vi "Convert Library and Other Files.vi"(8 "error in":errorcluster, 9 "main module path":path, 10 "project:open":refnum<vi>, 11 "dependency list[]":path[](array[path])) -> (0 "error out":errorcluster, 2 "outside vis":string[](array[string]), 3 "destination directory":path)   [LabVIEW 2021, in "Converter.lvlib"]
uses:
  Converter.lvlib
  TypeDefs/Library Data.ctl
  Converter Reusables/Converter Reusables.lvlib
  Path Functions/Path Functions.lvlib
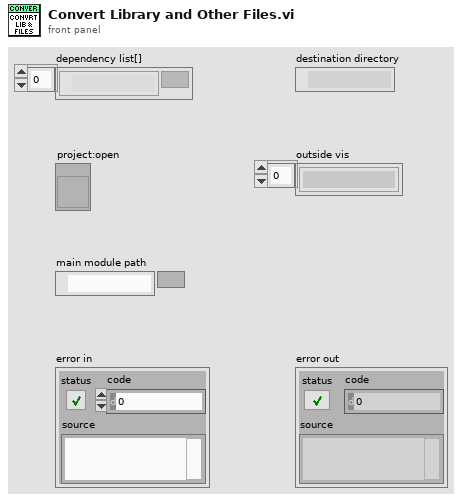
[diagram p1: front panel]
types:
  T1 = typedef "Converter.lvlib/Library Data.ctl" = cluster{"lib path":path, "lib name":string}
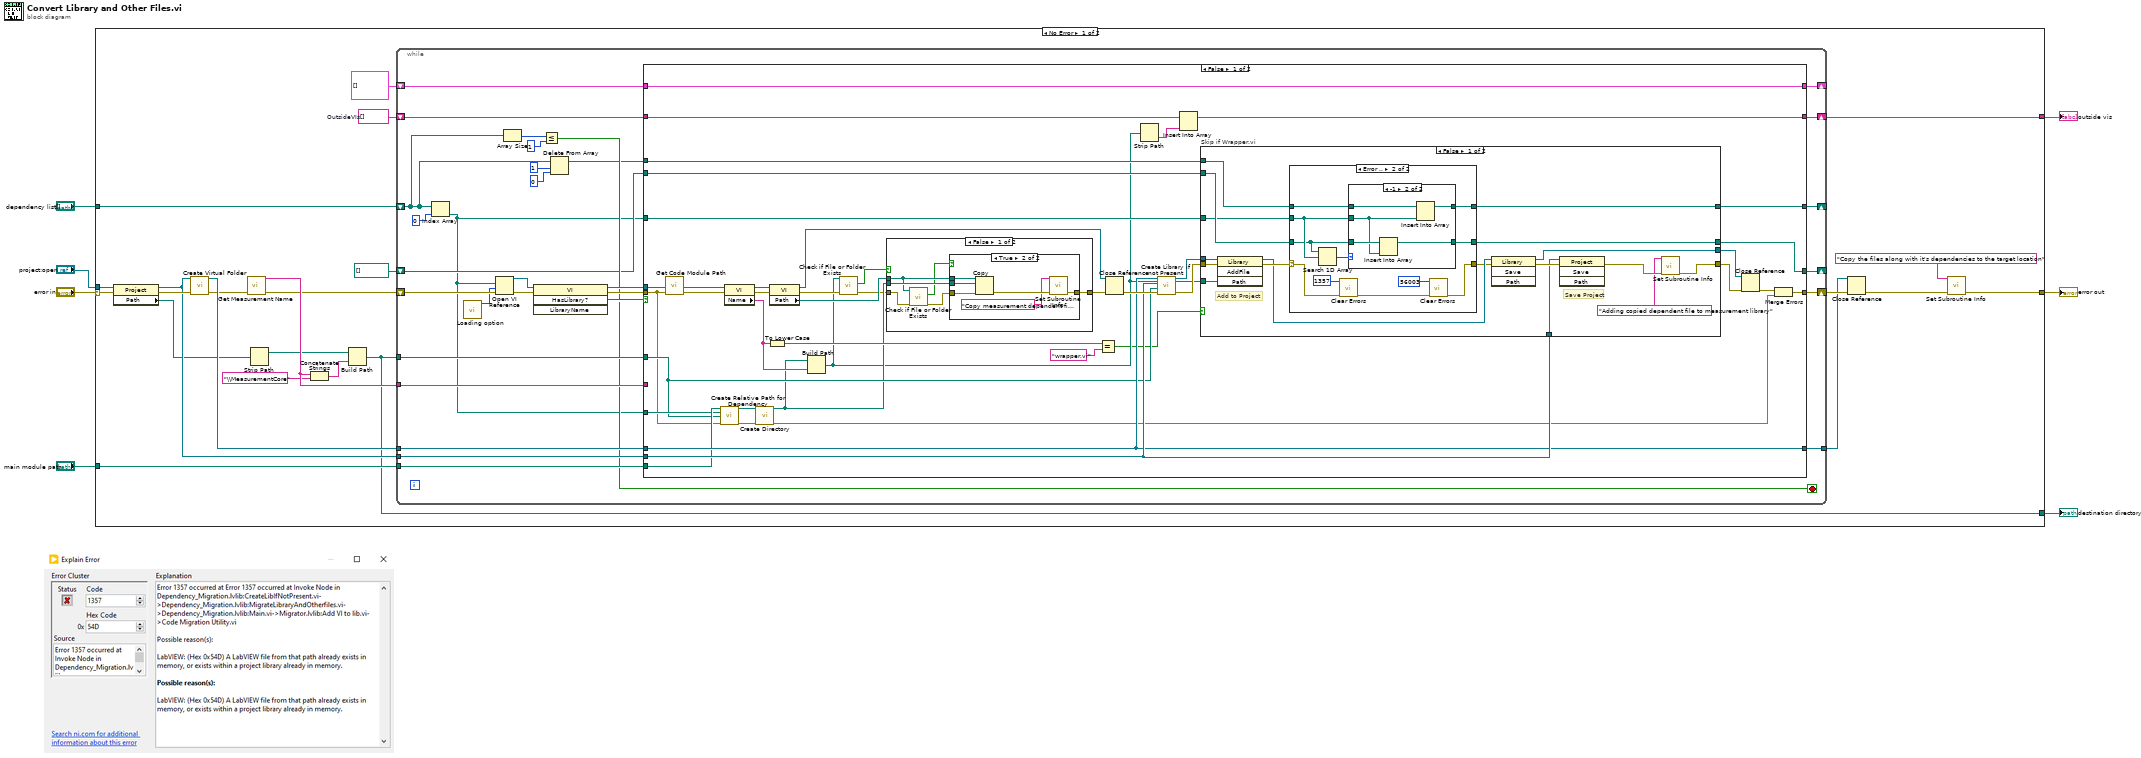
[diagram p0: block diagram]
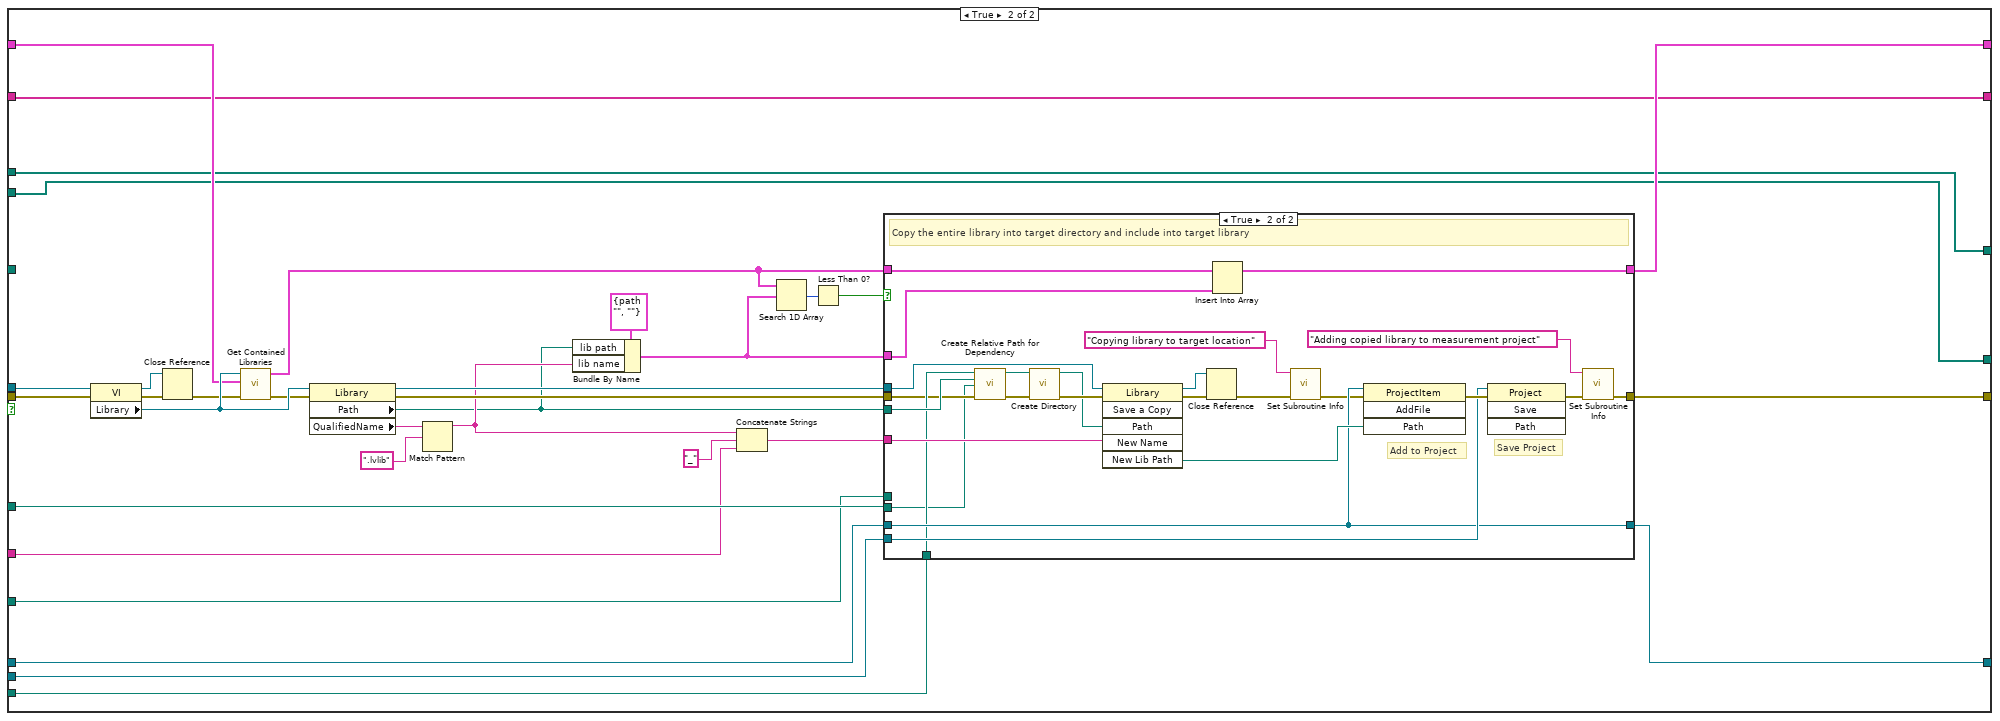
[diagram p7: hidden frame]
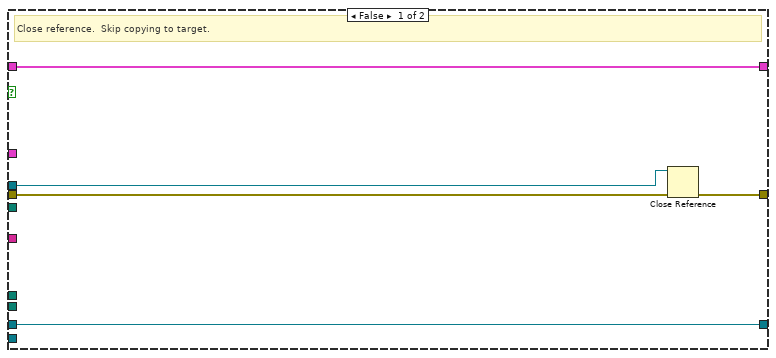
[diagram p8: hidden frame]
diagram:
  n1 = case shown="No Error" "error in" {
    selector: "error in" -> [w28 w222]
    tunnel: "project:open" -> [w29 _]
    tunnel: [w23 _] -> w5
    tunnel: "main module path" -> [w21 _]
    tunnel: [w15 _] -> w3
    tunnel: "dependency list[]" -> [w12 _]
    tunnel: [w9 w222] -> w1
    frame No Error {
      w24 = string[] []  # OutsideVIs
      n2 = property class="Project"(reference=w29, error in=w28) -> (reference out=w25:refnum<vi>, error out=w27:errorcluster, "Path"=w20:path)
      n3 = call "Create Virtual Folder.vi"("error in"=w27, "project in"=w25) -> ("error out"=w14:errorcluster, "virtual folder ref[]"=w26:refnum<vi>)  [unwired: 8 in]
      n4 = call "Get Measurement Name.vi"("error in"=w14) -> ("name out"=w19:string, "error out"=w13:errorcluster)  [unwired: 13 in]
      n5 = Strip Path(path=w20) -> (stripped path=w16:path)  [unwired: 1 out]
      n6 = Concatenate Strings(w19, "\\MeasurementCore") -> (w17:string)
      n7 = Build Path(base path=w16, name or relative path=w17) -> (appended path=w15:path)
      n8 = while {
        shift-right: [w55] -> _
        shift-left: T1[] [] ("Array") -> [w57]
        tunnel: w26 -> [w52]
        tunnel: w25 -> [w51]
        shift-right: [w49] -> w23
        shift-left: w24 -> [w50]
        tunnel: [w48] -> w22
        tunnel: w21 -> [w47]
        shift-right: [w56] -> w31
        shift-left: w13 -> [w54]
        tunnel: w19 -> [w46]
        tunnel: w15 -> [w45]
        shift-right: [w39] -> _
        shift-left: w12 -> [w32]
        shift-right: [w37] -> _
        shift-left: path[] [] -> [w38]
        stop <- w42 stop-if-true
        n9 = Index Array(array=w32, index=0) -> (element=w33:path)
        n10 = call "Loading option.vi"() -> ("options"=w35:i32)  [unwired: 11 in]
        n11 = Open VI Reference(vi path=w33, options=w35, error in (no error)=w54) -> (vi reference=w59:refnum<vi>, error out=w61:errorcluster)  [unwired: 3 in]
        n12 = Array Size(array=w32) -> (size(s)=w44:i32)
        n13 = invoke class="VI" method="HasLibrary?"(reference=w59, error in=w61) -> (reference out=w58:refnum<vi>, error out=w60:errorcluster, "Has Library?"=w53:bool)  [unwired: 2 in, 1 out]
        n14 = Less Or Equal?(x=w44, y=1) -> (x <= y?=w42:bool)
        n15 = Delete From Array(array=w32, length=1, index=0) -> (array with subset deleted=w40:path[])  [unwired: 1 out]
        n16 = case shown="False" w53 {
          tunnel: w60 -> [w76 w191]
          tunnel: w58 -> [w100 w190]
          tunnel: w45 -> [w77 w176]
          tunnel: w57 -> [w102 w180]
          tunnel: [w62 w184] -> w56
          tunnel: [w102 w183] -> w55
          tunnel: w52 -> [w87 w175]
          tunnel: w51 -> [w89 w167]
          tunnel: w50 -> [w94 w174]
          tunnel: [w93 w174] -> w49
          tunnel: [w87 w173] -> w48
          tunnel: w46 -> [_ w161]
          tunnel: w47 -> [w82 w171]
          tunnel: w33 -> [w81 w170]
          tunnel: w40 -> [w74 w169]
          tunnel: [w73 w169] -> w39
          tunnel: w33 -> [w72 _]
          tunnel: w38 -> [w68 w168]
          tunnel: [w67 w168] -> w37
          frame False {
            n17 = call "Get Code Module Path.vi"("error in"=w76) -> ("error out"=w75:errorcluster)  [unwired: 13 in, 1 out]
            n18 = call "Create Relative Path for Dependency.vi"("old main path"=w82, "old dependency path"=w81, "new dir"=w77, "error in"=w76) -> ("directory"=w79:path, "error out"=w80:errorcluster)  [unwired: 10 in]
            n19 = property class="VI"(reference=w100, error in=w75) -> (reference out=w99:refnum<vi>, error out=w101:errorcluster, "Name"=w84:string)
            n20 = call "Create Directory.vi"("directory"=w79, "error in"=w80) -> ("dup directory"=w71:path, "error out"=w78:errorcluster)  [unwired: 12 in]
            n21 = To Lower Case(string=w84) -> (all lower case string=w83:string)
            n22 = property class="VI"(reference=w99, error in=w101) -> (reference out=w96:refnum<vi>, error out=w70:errorcluster, "Path"=w97:path)
            n23 = Build Path(base path=w71, name or relative path=w84) -> (appended path=w66:path)
            n24 = call <vilib>:"Check if File or Folder Exists.vi"("error in (no error)"=w70, "path"=w66) -> ("error out"=w65:errorcluster, "file or folder exists?"=w69:bool)  [unwired: 7 in, 1 out]
            n25 = case shown="False" w69 {
              tunnel: [w107 w116] -> w98
              tunnel: w97 -> [w106 _]
              tunnel: w71 -> [w108 _]
              tunnel: w65 -> [w103 w116]
              frame False {
                n26 = call <vilib>:"Check if File or Folder Exists.vi"("error in (no error)"=w103, "path"=w106) -> ("error out"=w105:errorcluster, "file or folder exists?"=w104:bool)  [unwired: 7 in, 1 out]
                n27 = case shown="True" w104 {
                  tunnel: w106 -> [_ w115]
                  tunnel: w108 -> [_ w114]
                  tunnel: w105 -> [w109 w113]
                  tunnel: [w109 w111] -> w107
                  frame False {
                  }
                  frame True {
                    n28 = Copy(8:w113, 10:w114, 11:w115) -> (0:w112:errorcluster)  [unwired: 2 in, 2 out]
                    n29 = call "Set Subroutine Info.vi"("subroutine in"="Copy measurement dependent file to measurement project location" ("Subroutine In"), "error in"=w112) -> ("error out"=w111:errorcluster)  [unwired: 13 in]
                  }
                }
              }
              frame True {
              }
            }
            n30 = Equal?(x=w83, y="wrapper.vi") -> (x = y?=w63:bool)
            n31 = Close Reference(reference=w96, error in (no error)=w98) -> (error out=w91:errorcluster)
            n32 = Strip Path(path=w66) -> (name=w92:string)  [unwired: 1 out]
            n33 = call "Create Library if not Present.vi"("error in"=w91, "dest directory"=w77, "project ref"=w89, "virtual folder ref"=w87) -> ("error out"=w90:errorcluster, "library refnum"=w88:refnum<vi>)  [unwired: 6 in]
            n34 = Insert Into Array(array=w94, new element=w92) -> (w93:string[])  [unwired: 1 in]
            n35 = case "Skip if Wrapper.vi" shown="False" w63 {
              tunnel: [w120 w158] -> w95
              tunnel: w66 -> [w132 _]
              tunnel: w90 -> [w131 w158]
              tunnel: w89 -> [w117 _]
              tunnel: w88 -> [w130 w157]
              tunnel: [w128 w157] -> w85
              tunnel: w74 -> [w125 w156]
              tunnel: [w124 w156] -> w73
              tunnel: w72 -> [w118 _]
              tunnel: w68 -> [w123 w155]
              tunnel: [w122 w155] -> w67
              frame False {
                # "Save Project"
                # "Add to Project"
                n36 = invoke class="Library" method="AddFile"(reference=w130, error in=w131, "Path"=w132) -> (reference out=w129:refnum<vi>, error out=w133:errorcluster)  [unwired: 1 in, 2 out]
                n37 = case shown="Error .." w133 {
                  selector: w133 -> [w135 w147]
                  tunnel: [w135 w143] -> w126
                  tunnel: w125 -> [w136 w142]
                  tunnel: [w136 w141] -> w124
                  tunnel: w118 -> [_ w139]
                  tunnel: w123 -> [w134 w137]
                  tunnel: [w134 w140] -> w122
                  frame No Error {
                  }
                  frame Error {
                    n38 = Search 1D Array(1D array=w137, element=w139) -> (index of element=w138:i32)  [unwired: 1 in]
                    n39 = call <vilib>:"Clear Errors.vi"("error in (no error)"=w147, "specific error code to clear (0: all)"=1357) -> ("error out"=w144:errorcluster)  [unwired: 4 in, 1 out]
                    n40 = case shown="-1" w138 {
                      tunnel: w142 -> [w149 w154]
                      tunnel: [w149 w153] -> w141
                      tunnel: [w148 w152] -> w140
                      tunnel: w137 -> [w148 w151]
                      tunnel: w139 -> [_ w150]
                      frame Default {
                      }
                      frame -1 {
                        n41 = Insert Into Array(array=w151, new element=w150) -> (w152:path[])  [unwired: 1 in]
                        n42 = Insert Into Array(array=w154, new element=w150) -> (w153:path[])  [unwired: 1 in]
                      }
                    }
                    n43 = call <vilib>:"Clear Errors.vi"("error in (no error)"=w144, "specific error code to clear (0: all)"=56003) -> ("error out"=w143:errorcluster)  [unwired: 4 in, 1 out]
                  }
                }
                n44 = invoke class="Library" method="Save"(reference=w129, error in=w126) -> (reference out=w128:refnum<vi>, error out=w127:errorcluster)  [unwired: 2 in, 2 out]
                n45 = invoke class="Project" method="Save"(reference=w117, error in=w127) -> (error out=w121:errorcluster)  [unwired: 2 in, 3 out]
                n46 = call "Set Subroutine Info.vi"("subroutine in"="Adding copied dependent file to measurement library" ("Subroutine In"), "error in"=w121) -> ("error out"=w120:errorcluster)  [unwired: 13 in]
              }
              frame True {
              }
            }
            n47 = Close Reference(reference=w85, error in (no error)=w95) -> (error out=w86:errorcluster)
            n48 = Merge Errors(w86, w78) -> (w62:errorcluster)
          }
          frame True {
            n49 = property class="VI"(reference=w190, error in=w191) -> (reference out=w182:refnum<vi>, error out=w189:errorcluster, "Library"=w181:refnum<vi>)
            n50 = Close Reference(reference=w182, error in (no error)=w189) -> (error out=w179:errorcluster)
            n51 = call "Get Contained Libraries.vi"("error in"=w179, "lib data in[]"=w180, "library in"=w181) -> ("error out"=w178:errorcluster, "lib data out[]"=w163:T1[])  [unwired: 7 in]
            n52 = property class="Library"(reference=w181, error in=w178) -> (reference out=w186:refnum<vi>, error out=w185:errorcluster, "Path"=w166:path, "QualifiedName"=w165:string)
            n53 = Match Pattern(string=w165, regular expression=".lvlib") -> (before substring=w172:string)  [unwired: 1 in, 3 out]
            n54 = Bundle By Name(cluster=T1 {"lib path"=path "", "lib name"=""}, "lib path"=w166, "lib name"=w172) -> (w162:T1)
            n55 = Concatenate Strings(w172, "_" ("string"), w161) -> (w177:string)
            n56 = Search 1D Array(1D array=w163, element=w162) -> (index of element=w188:i32)  [unwired: 1 in]
            n57 = Less Than 0?(x=w188) -> (x < 0?=w187:bool)
            n58 = case shown="True" w187 {
              tunnel: w162 -> [_ w219]
              tunnel: w163 -> [w196 w220]
              tunnel: [w196 w221] -> w183
              tunnel: w185 -> [w193 w206]
              tunnel: w186 -> [w194 w218]
              tunnel: [w195 w201] -> w184
              tunnel: w176 -> [_ w203]
              tunnel: w177 -> [_ w214]
              tunnel: w175 -> [w192 w211]
              tunnel: w167 -> [_ w212]
              tunnel: [w192 w211] -> w173
              tunnel: w166 -> [_ w210]
              tunnel: w171 -> [_ w209]
              tunnel: w170 -> [_ _]
              frame False {
                # "Close reference.  Skip copying to target."
                n59 = Close Reference(reference=w194, error in (no error)=w193) -> (error out=w195:errorcluster)
              }
              frame True {
                # "Save Project"
                # "Add to Project"
                # "Copy the entire library into target directory and include into target library"
                n60 = call "Create Relative Path for Dependency.vi"("old main path"=w209, "old dependency path"=w210, "new dir"=w203, "error in"=w206) -> ("directory"=w208:path, "error out"=w207:errorcluster)  [unwired: 10 in]
                n61 = call "Create Directory.vi"("directory"=w208, "error in"=w207) -> ("dup directory"=w204:path, "error out"=w205:errorcluster)  [unwired: 12 in]
                n62 = invoke class="Library" method="Save a Copy"(reference=w218, error in=w205, "Path"=w204, "New Name"=w214) -> (reference out=w215:refnum<vi>, error out=w216:errorcluster, "New Lib Path"=w213:path)  [unwired: 2 in, 3 out]
                n63 = Close Reference(reference=w215, error in (no error)=w216) -> (error out=w199:errorcluster)
                n64 = Insert Into Array(array=w220, new element=w219) -> (w221:T1[])  [unwired: 1 in]
                n65 = call "Set Subroutine Info.vi"("subroutine in"="Copying library to target location" ("Subroutine In"), "error in"=w199) -> ("error out"=w198:errorcluster)  [unwired: 13 in]
                n66 = invoke class="ProjectItem" method="AddFile"(reference=w211, error in=w198, "Path"=w213) -> (error out=w217:errorcluster)  [unwired: 1 in, 3 out]
                n67 = invoke class="Project" method="Save"(reference=w212, error in=w217) -> (error out=w202:errorcluster)  [unwired: 2 in, 3 out]
                n68 = call "Set Subroutine Info.vi"("subroutine in"="Adding copied library to measurement project" ("Subroutine In"), "error in"=w202) -> ("error out"=w201:errorcluster)  [unwired: 13 in]
              }
            }
          }
        }
      }
      n69 = Close Reference(reference=w22, error in (no error)=w31) -> (error out=w10:errorcluster)
      n70 = call "Set Subroutine Info.vi"("subroutine in"="Copy the files along with it's dependencies to the target location" ("Subroutine In"), "error in"=w10) -> ("error out"=w9:errorcluster)  [unwired: 13 in]
    }
    frame Error {
    }
  }
  "error out" <- w1
  "destination directory" <- w3
  "outside vis" <- w5
